vi "Distance Between Particles.vi"(11 "Particle Reports":T2(array[cluster]) {"Orientation" format="%.2f"; "Dimensions"."Height" format="%.2f"; "Dimensions"."Width" format="%.2f"; "Center of Mass"."Y" format="%.2f"; "Center of Mass"."X" format="%.2f"; "Bounding Rect"."Bottom" format="%.2f"; "Bounding Rect"."Right" format="%.2f"; "Bounding Rect"."Top" format="%.2f"; "Bounding Rect"."Left" format="%.2f"; "Number of Holes" format="%.2f"; "Area" format="%.2f"}) -> (3 "output array":T1(array[cluster]))   [LabVIEW 2011]
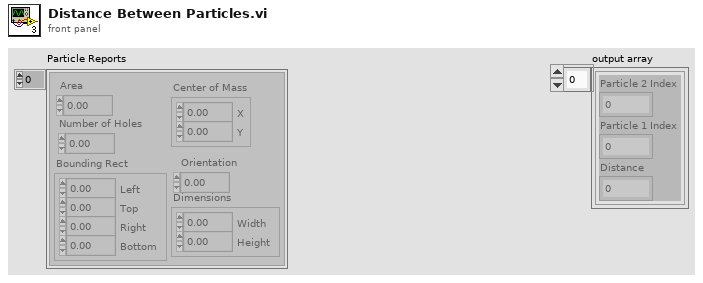
[diagram p1: front panel]
types:
  T1 = cluster{"Particle 2 Index":i32, "Particle 1 Index":i32, "Distance":dbl}[]
  T2 = cluster{"Area":dbl, "Number of Holes":dbl, "Bounding Rect":cluster{"Left":dbl, "Top":dbl, "Right":dbl, "Bottom":dbl}, "Center of Mass":cluster{"X":dbl, "Y":dbl}, "Orientation":dbl, "Dimensions":cluster{"Width":dbl, "Height":dbl}}[]
  T3 = cluster{"Particle 2 Index":i32, "Particle 1 Index":i32, "Distance":dbl}
  T4 = cluster{"Area":dbl, "Number of Holes":dbl, "Bounding Rect":cluster{"Left":dbl, "Top":dbl, "Right":dbl, "Bottom":dbl}, "Center of Mass":cluster{"X":dbl, "Y":dbl}, "Orientation":dbl, "Dimensions":cluster{"Width":dbl, "Height":dbl}}
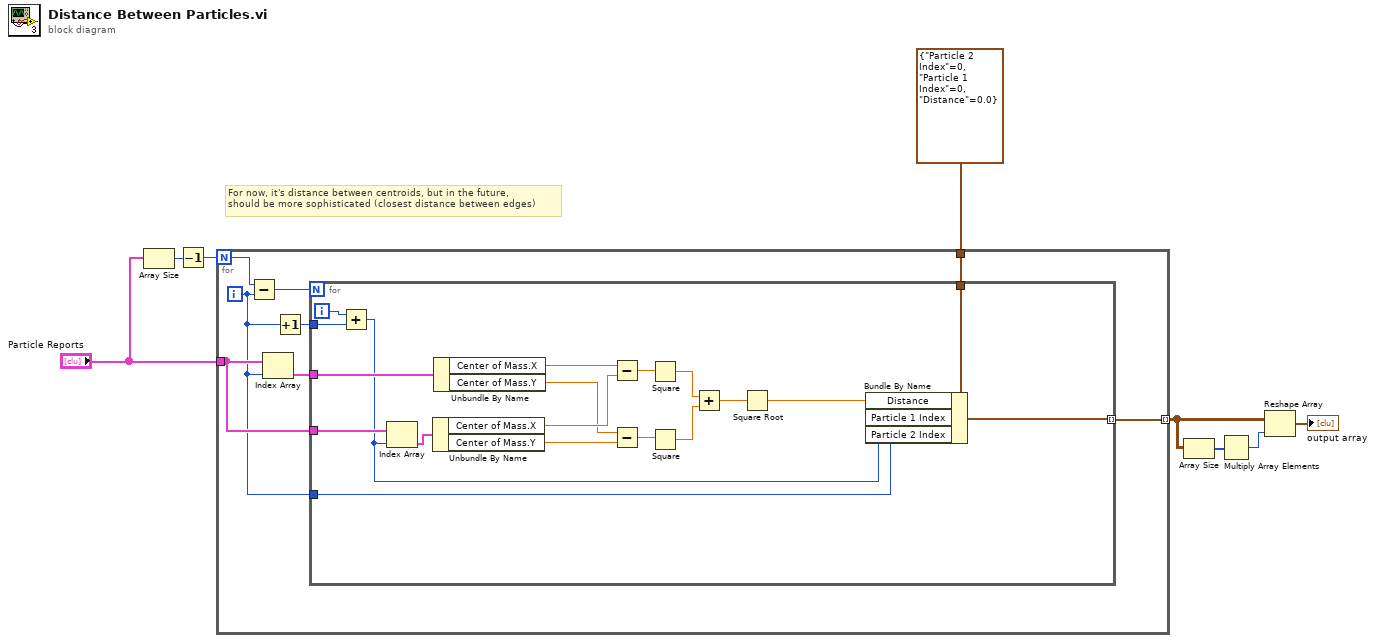
[diagram p0: block diagram]
diagram:
  # "For now, it's distance between centroids, but in the future, \nshould be more sophisticated (closest distance between edges)"
  n1 = Array Size(array="Particle Reports") -> (size(s)=w2:i32)
  n2 = Decrement(x=w2) -> (x-1=w3:i32)
  n3 = for {
    N: w3 -> [w16]
    tunnel: "Particle Reports" -> [w14]
    tunnel: [w12] -> w7 mode=indexing
    tunnel: T3 {"Particle 2 Index"=0, "Particle 1 Index"=0, "Distance"=0.0} ("input cluster") -> [w10]
    i -> [w11]
    n4 = Subtract(x=w16, y=w11) -> (x-y=w9:i32)
    n5 = Index Array(array=w14, index=w11) -> (element=w13:T4)
    n6 = Increment(x=w11) -> (x+1=w15:i32)
    n7 = for {
      N: w9 -> [_]
      tunnel: w15 -> [w34]
      tunnel: w14 -> [w33]
      tunnel: w13 -> [w31]
      tunnel: [w17] -> w12 mode=indexing
      tunnel: w11 -> [w20]
      tunnel: w10 -> [w18]
      i -> [w35]
      n8 = Add(x=w35, y=w34) -> (x+y=w19:i32)
      n9 = Index Array(array=w33, index=w19) -> (element=w32:T4)
      n10 = Unbundle By Name(w32) -> ("Center of Mass.X"=w28:dbl, "Center of Mass.Y"=w26:dbl)
      n11 = Unbundle By Name(w31) -> ("Center of Mass.X"=w29:dbl, "Center of Mass.Y"=w27:dbl)
      n12 = Subtract(x=w29, y=w28) -> (x-y=w25:dbl)
      n13 = Subtract(x=w27, y=w26) -> (x-y=w24:dbl)
      n14 = Square(x=w25) -> (x^2=w23:dbl)
      n15 = Square(x=w24) -> (x^2=w22:dbl)
      n16 = Add(x=w23, y=w22) -> (x+y=w30:dbl)
      n17 = Square Root(x=w30) -> (sqrt(x)=w21:dbl)
      n18 = Bundle By Name(cluster=w18, "Distance"=w21, "Particle 1 Index"=w19, "Particle 2 Index"=w20) -> (w17:T3)
    }
  }
  n19 = Array Size(array=w7) -> (size(s)=w6:i32[])
  n20 = Multiply Array Elements(1:w6) -> (0:w5:i32)
  n21 = Reshape Array(w7, w5) -> (→"output array":T1)
